vi "Error_Info.vi"(8 "error in (no error)":errorcluster, 10 "errorcode":i32, 11 "tag handle":i32) -> (0 "error out":errorcluster, 2 "error description":string, 3 "tag handle out":i32)   [LabVIEW 2016]
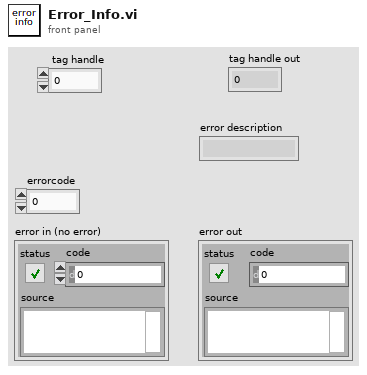
[diagram p1: front panel]
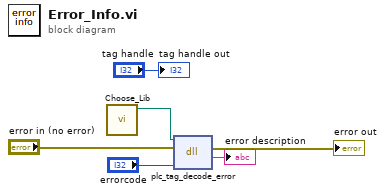
[diagram p0: block diagram]
diagram:
  n1 = call "Choose_Lib.vi"() -> ("appended path"=w1:path)  [unwired: 11 in]
  n2 = dll-call lib="?" fn="plc_tag_decode_error"(path in=w1, error in="error in (no error)", "errorcode"="errorcode") -> (error out=→"error out":errorcluster, "return type"=→"error description":string)  [unwired: 2 in, 1 out]
  "tag handle out" <- "tag handle"
